vi "9759 RevB Write.vi"(5 "Settings.ControlCals":T2(array[cluster]), 6 "Device Inputs":dbl[](array[numeric]), 7 "FIFO Indexes.Write":T3, 8 "error in":errorcluster, 9 "dt (sec)":sgl, 10 "Data":T1, 11 "FPGA Ref in":T4) -> (0 "error out":errorcluster, 3 "FPGA Ref out":T4)   [LabVIEW 2015, in "NI 9759 RevB Custom Device.lvlib"]
uses:
  NI 9759 RevB Custom Device.lvlib
  Shared/Types/9759 RevB FPGA Ref.ctl
  <vilib>/Utility/error.llb/Error Cluster From Error Code.vi
  <vilib>/rvi/errors/niLvFpgaAdjustHostInterfaceError.vi
  <vilib>/rvi/interface/nirviReadWriteControl/nirviReadWriteControl.xnode
  NiFpgaLv.dll
  <vilib>/rvi/interface/Simulation/niFpgaSimulationCallBeginRW.vi
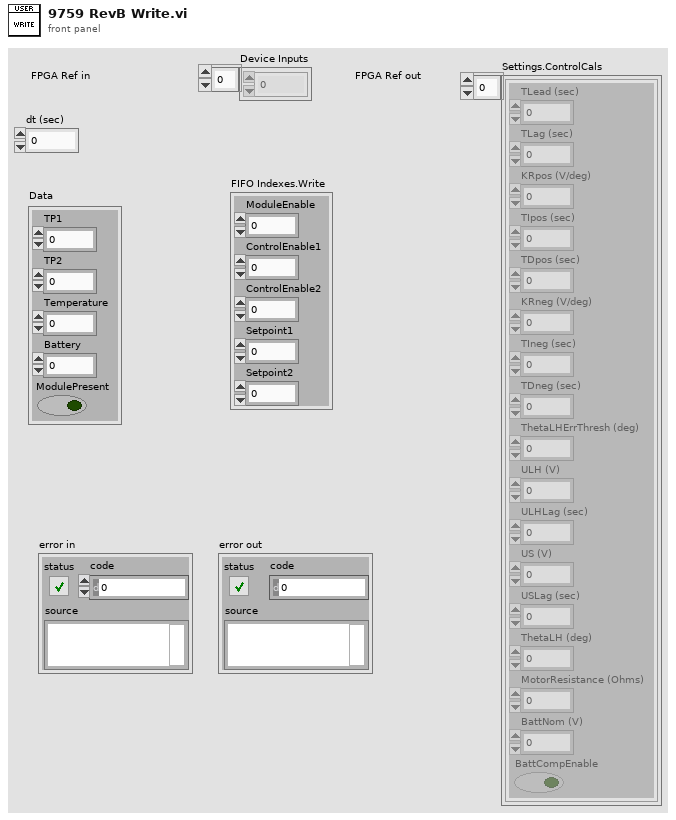
[diagram p1: front panel]
types:
  T1 = cluster{"TP1":sgl, "TP2":sgl, "Temperature":sgl, "Battery":sgl, "ModulePresent":bool}
  T2 = cluster{"TLead (sec)":sgl, "TLag (sec)":sgl, "KRpos (V/deg)":sgl, "TIpos (sec)":sgl, "TDpos (sec)":sgl, "KRneg (V/deg)":sgl, "TIneg (sec)":sgl, "TDneg (sec)":sgl, "ThetaLHErrThresh (deg)":sgl, "ULH (V)":sgl, "ULHLag (sec)":sgl, "US (V)":sgl, "USLag (sec)":sgl, "ThetaLH (deg)":sgl, "MotorResistance (Ohms)":sgl, "BattNom (V)":sgl, "BattCompEnable":bool}[]
  T3 = cluster{"ModuleEnable":i32, "ControlEnable1":i32, "ControlEnable2":i32, "Setpoint1":i32, "Setpoint2":i32}
  T4 = typedef "NI 9759 RevB Custom Device.lvlib/9759 RevB FPGA Ref.ctl" = refnum<k20>
  T5 = cluster{"ModuleEnable":bool, "WatchdogIn":bool, "Throttle1Period":u16, "Throttle2Period":u16, "Throttle1PulseWidth":i16, "Throttle2PulseWidth":i16}
  T6 = cluster{"TLead (sec)":sgl, "TLag (sec)":sgl, "KRpos (V/deg)":sgl, "TIpos (sec)":sgl, "TDpos (sec)":sgl, "KRneg (V/deg)":sgl, "TIneg (sec)":sgl, "TDneg (sec)":sgl, "ThetaLHErrThresh (deg)":sgl, "ULH (V)":sgl, "ULHLag (sec)":sgl, "US (V)":sgl, "USLag (sec)":sgl, "ThetaLH (deg)":sgl, "MotorResistance (Ohms)":sgl, "BattNom (V)":sgl, "BattCompEnable":bool}
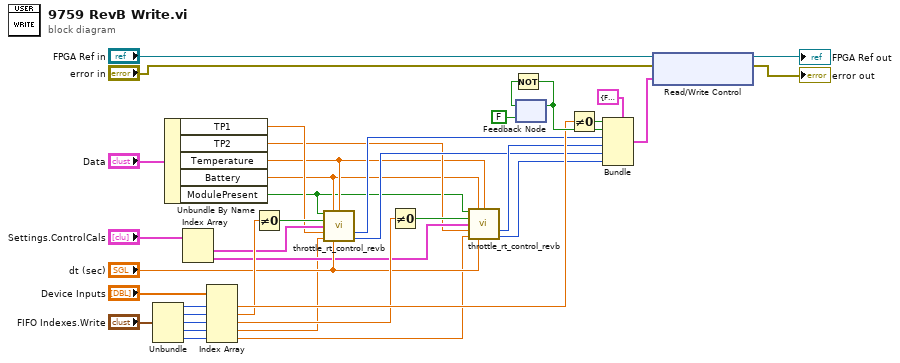
[diagram p0: block diagram]
diagram:
  n1 = Unbundle("FIFO Indexes.Write") -> ("ModuleEnable"=w32:i32, "ControlEnable1"=w31:i32, "ControlEnable2"=w30:i32, "Setpoint1"=w29:i32, "Setpoint2"=w28:i32)
  n2 = Unbundle By Name("Data") -> ("TP1"=w5:sgl, "TP2"=w4:sgl, "Temperature"=w3:sgl, "Battery"=w2:sgl, "ModulePresent"=w1:bool)
  n3 = Index Array(array="Settings.ControlCals") -> (element #1=w10:T6, element #2=w9:T6)  [unwired: 2 in]
  n4 = Index Array(array="Device Inputs", index #1=w32, index #2=w31, index #3=w30, index #4=w29, index #5=w28) -> (element #1=w21:dbl, element #2=w15:dbl, element #3=w12:dbl, element #4=w8:dbl, element #5=w7:dbl)
  n5 = Not Equal To 0?(x=w15) -> (x != 0?=w14:bool)
  n6 = call <vilib>:"throttle_rt_control_revb.vi"("ModulePresent"=w1, "Battery (V)"=w2, "Temperature (C)"=w3, "ControlEnable"=w14, "ThrottleCalibrations"=w10, "Theta (deg)"=w5, "ThetaR (deg)"=w8, "dt (sec)"="dt (sec)") -> ("ThrottlePeriodTicks"=w18:u16, "ThrottlePulseWidthTicks"=w17:i16)  [unwired: 5 in, 1 out]
  n7 = Not Equal To 0?(x=w12) -> (x != 0?=w13:bool)
  n8 = call <vilib>:"throttle_rt_control_revb.vi"("ModulePresent"=w1, "Battery (V)"=w2, "Temperature (C)"=w3, "ControlEnable"=w13, "ThrottleCalibrations"=w9, "Theta (deg)"=w4, "ThetaR (deg)"=w7, "dt (sec)"="dt (sec)") -> ("ThrottlePeriodTicks"=w19:u16, "ThrottlePulseWidthTicks"=w16:i16)  [unwired: 5 in, 1 out]
  n9 = feedback #1(FALSE) -> (w24:bool)
  n10 = Not(x=w24) -> (.not. x?=w22:bool)
  n11 = feedback-in #1(w22) -> ()
  n12 = Not Equal To 0?(x=w21) -> (x != 0?=w20:bool)
  n13 = Bundle(cluster=T5 {"ModuleEnable"=FALSE, "WatchdogIn"=FALSE, "Throttle1Period"=0, "Throttle2Period"=0, "Throttle1PulseWidth"=0, "Throttle2PulseWidth"=0} ("ThrottleControl"), "ModuleEnable"=w20, "WatchdogIn"=w22, "Throttle1Period"=w18, "Throttle2Period"=w19, "Throttle1PulseWidth"=w17, "Throttle2PulseWidth"=w16) -> (w25:T5)
  n14 = xnode "Read/Write Control"("FPGA VI Reference In"="FPGA Ref in", "error in"="error in", "ThrottleControl"=w25) -> ("FPGA VI Reference Out"=→"FPGA Ref out":T4, "error out"=→"error out":errorcluster)
